vi "clean up tag removing module.vi"(10 "module ID":string, 11 "Tag Info in":T1) -> (3 "Tag Info out":T1)   [LabVIEW 2013, in "engine configuration.lvclass"]
uses:
  engine configuration.lvclass
  Tag Info.ctl
  <vilib>/NI/Tag Bus/tag/tag descriptor.lvclass
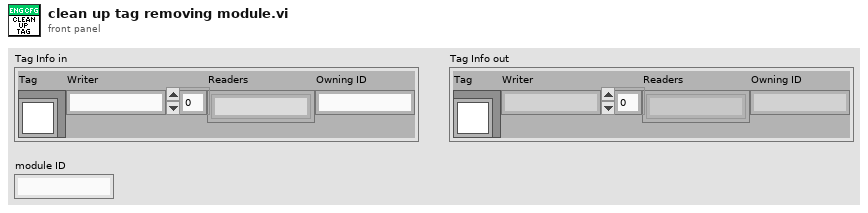
[diagram p1: front panel]
types:
  T1 = typedef "engine configuration.lvclass/Tag Info.ctl" = cluster{"Tag":refnum<class "tag descriptor.lvclass">, "Writer":string, "Readers":string[], "Owning ID":string}
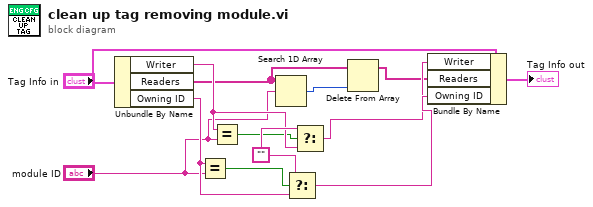
[diagram p0: block diagram]
diagram:
  w12 = ""
  n1 = Unbundle By Name("Tag Info in") -> ("Writer"=w8:string, "Readers"=w4:string[], "Owning ID"=w11:string)
  n2 = Equal?(x=w11, y="module ID") -> (x = y?=w10:bool)
  n3 = Equal?(x=w8, y="module ID") -> (x = y?=w7:bool)
  n4 = Search 1D Array(1D array=w4, element="module ID") -> (index of element=w5:i32)  [unwired: 1 in]
  n5 = Select(t=w12, s=w10, f=w11) -> (s? t:f=w13:string)
  n6 = Select(t=w12, s=w7, f=w8) -> (s? t:f=w9:string)
  n7 = Delete From Array(array=w4, index=w5) -> (array with subset deleted=w6:string[])  [unwired: 1 in, 1 out]
  n8 = Bundle By Name(cluster="Tag Info in", "Writer"=w9, "Readers"=w6, "Owning ID"=w13) -> (→"Tag Info out":T1)
